vi "S1.vi"(1 "Input array":bool[](array[boolean])) -> (0 "Array":bool[](array[boolean]))   [LabVIEW 2013]
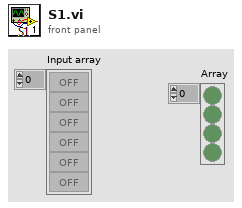
[diagram p1: front panel]
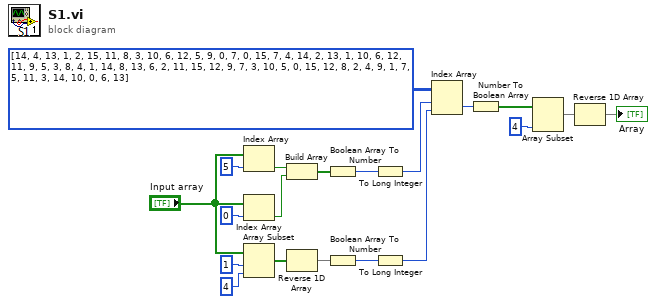
[diagram p0: block diagram]
diagram:
  n1 = Index Array(array="Input array", index=5) -> (element=w3:bool)
  n2 = Index Array(array="Input array", index=0) -> (element=w2:bool)
  n3 = Array Subset(array="Input array", index=1, length=4) -> (w5:bool[])
  n4 = Build Array(w3, w2) -> (w1:bool[])
  n5 = Reverse 1D Array(array=w5) -> (reversed array=w4:bool[])
  n6 = Boolean Array To Number(Boolean array=w1) -> (number=w12:u32)
  n7 = Boolean Array To Number(Boolean array=w4) -> (number=w11:u32)
  n8 = To Long Integer(number=w12) -> (32bit integer=w9:i32)
  n9 = To Long Integer(number=w11) -> (32bit integer=w10:i32)
  n10 = Index Array(array=u8[][] [[14, 4, 13, 1, 2, 15, 11, 8, 3, 10, 6, 12, 5, 9, 0, 7], [0, 15, 7, 4, 14, 2, 13, 1, 10, 6, 12, 11, 9, 5, 3, 8], [4, 1, 14, 8, 13, 6, 2, 11, 15, 12, 9, 7, 3, 10, 5, 0], [15, 12, 8, 2, 4, 9, 1, 7, 5, 11, 3, 14, 10, 0, 6, 13]], index (row)=w9, index (col)=w10) -> (element=w15:u8)
  n11 = Number To Boolean Array(number=w15) -> (Boolean array=w14:bool[])
  n12 = Array Subset(array=w14, length=4) -> (w6:bool[])  [unwired: 1 in]
  n13 = Reverse 1D Array(array=w6) -> (reversed array=→"Array":bool[])
